vi "dispense off.vi"(6 "dispense status data IN":T1, 8 "error in":errorcluster, 9 "dispense run off":bool, 10 "dispense in":T2={"Vacuum Setting (0000)"=0, "Pressure"=20, "on delay (ms)"=0.5, "off delay (ms) "=0.5} {"Vacuum Setting (0000)" min=0 max=1000 step=1 format="%04.0f"}, 11 "Ultimus V2.lvclass":refnum<class "Ultimus V2.lvclass">) -> (0 "error out":errorcluster, 2 "dispense out":T2={"Vacuum Setting (0000)"=0, "Pressure"=20, "on delay (ms)"=0.5, "off delay (ms) "=0.5} {"Vacuum Setting (0000)" min=0 max=1000 step=1 format="%04.0f"}, 3 "Ultimus V2.lvclass 2":refnum<class "Ultimus V2.lvclass">, 4 "dispense status data OUT":T1)   [LabVIEW 2016]
uses:
  Classes/Controller/Dispenser/Ultimus V2 Folder/Ultimus V2.lvclass
  dispense status data.ctl
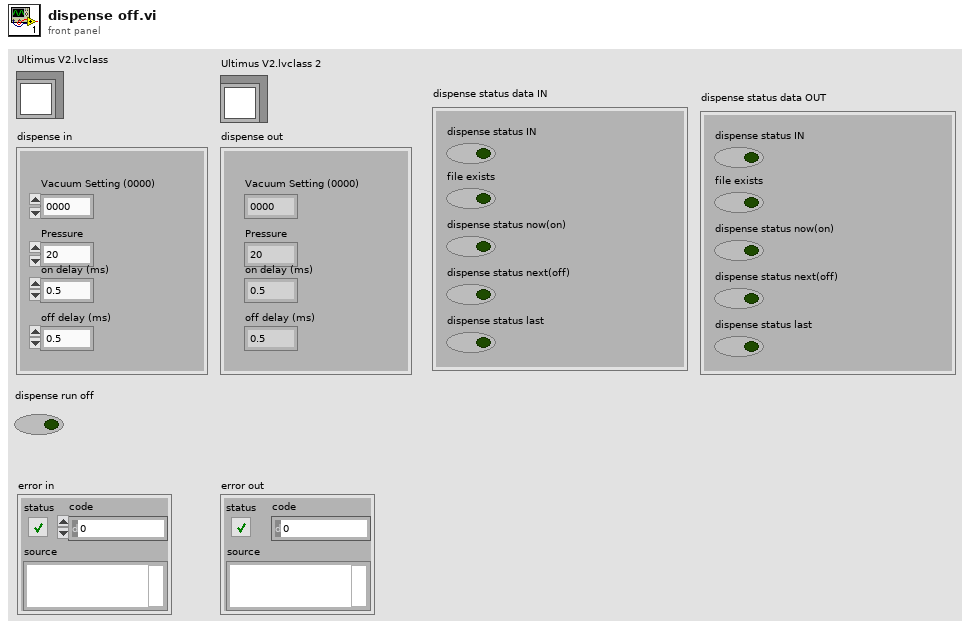
[diagram p1: front panel]
types:
  T1 = typedef "dispense status data.ctl" = cluster{"file exists":bool, "dispense status now(on)":bool, "dispense status next(off)":bool, "dispense status IN":bool, "dispense status last":bool}
  T2 = cluster{"Vacuum Setting (0000)":i64, "Pressure":i16, "on delay (ms)":dbl, "off delay (ms) ":dbl}
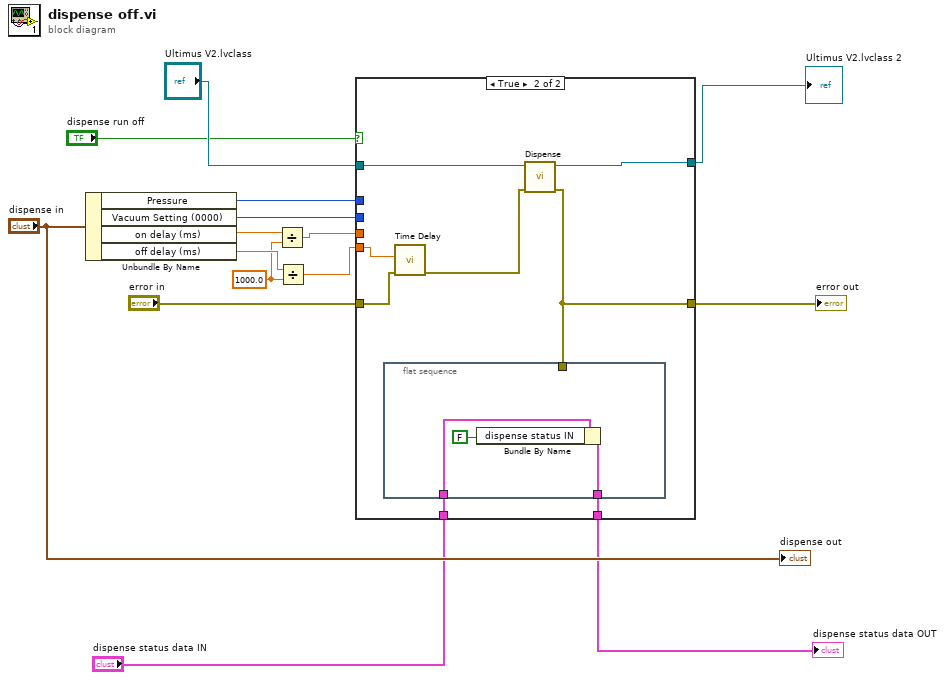
[diagram p0: block diagram]
diagram:
  w3 = 1000.0 ("y")
  n1 = Unbundle By Name("dispense in") -> ("Pressure"=w12:i16, "Vacuum Setting (0000)"=w11:i64, "on delay (ms)"=w4:dbl, "off delay (ms)"=w6:dbl)
  n2 = Divide(x=w4, y=w3) -> (x/y=w5:dbl)
  n3 = Divide(x=w6, y=w3) -> (x/y=w7:dbl)
  n4 = case shown="True" "dispense run off" {
    tunnel: [w18 w25] -> w14
    tunnel: "Ultimus V2.lvclass" -> [w18 w24]
    tunnel: [w17 w21] -> w10
    tunnel: w11 -> [_ _]
    tunnel: w12 -> [_ _]
    tunnel: w5 -> [_ _]
    tunnel: "error in" -> [w17 w22]
    tunnel: w7 -> [_ w26]
    tunnel: "dispense status data IN" -> [w16 w20]
    tunnel: [w16 w19] -> w1
    frame False {
    }
    frame True {
      n5 = flat-sequence {
        tunnel: w21 -> [_]
        tunnel: w20 -> [w29]
        tunnel: [w27] -> w19
        frame #0 {
          n6 = Bundle By Name(cluster=w29, "dispense status IN"=FALSE ("file exists")) -> (w27:T1)
        }
      }
      n7 = call "Time Delay"("error in (no error)"=w22, "Delay Time (s)"=w26) -> ("error out"=w23:errorcluster)  [unwired: 9 in]
      n8 = call-dynamic "Dispense.vi"("error in (no error)"=w23, "Ultimus V in"=w24) -> ("error out"=w21:errorcluster, "Ultimus V out"=w25:refnum<class "Ultimus V2.lvclass">)  [unwired: 8 in]
    }
  }
  "Ultimus V2.lvclass 2" <- w14
  "error out" <- w10
  "dispense status data OUT" <- w1
  "dispense out" <- "dispense in"
